vi "switch_load_1.vi"(0 "Node":string, 1 "event time":string="0.023560", 2 "Event type":string="BCG") -> (7 "Event switches":string caption="Result")   [LabVIEW 2019]
panel:
  in  "Evento?":bool
  # "CHAVEIA CARGAS DO SISTEMA"
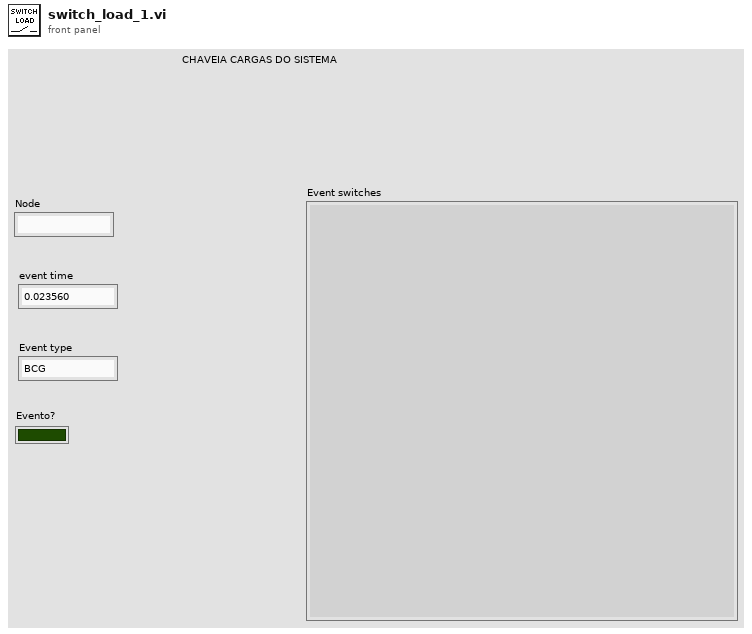
[diagram p1: front panel]
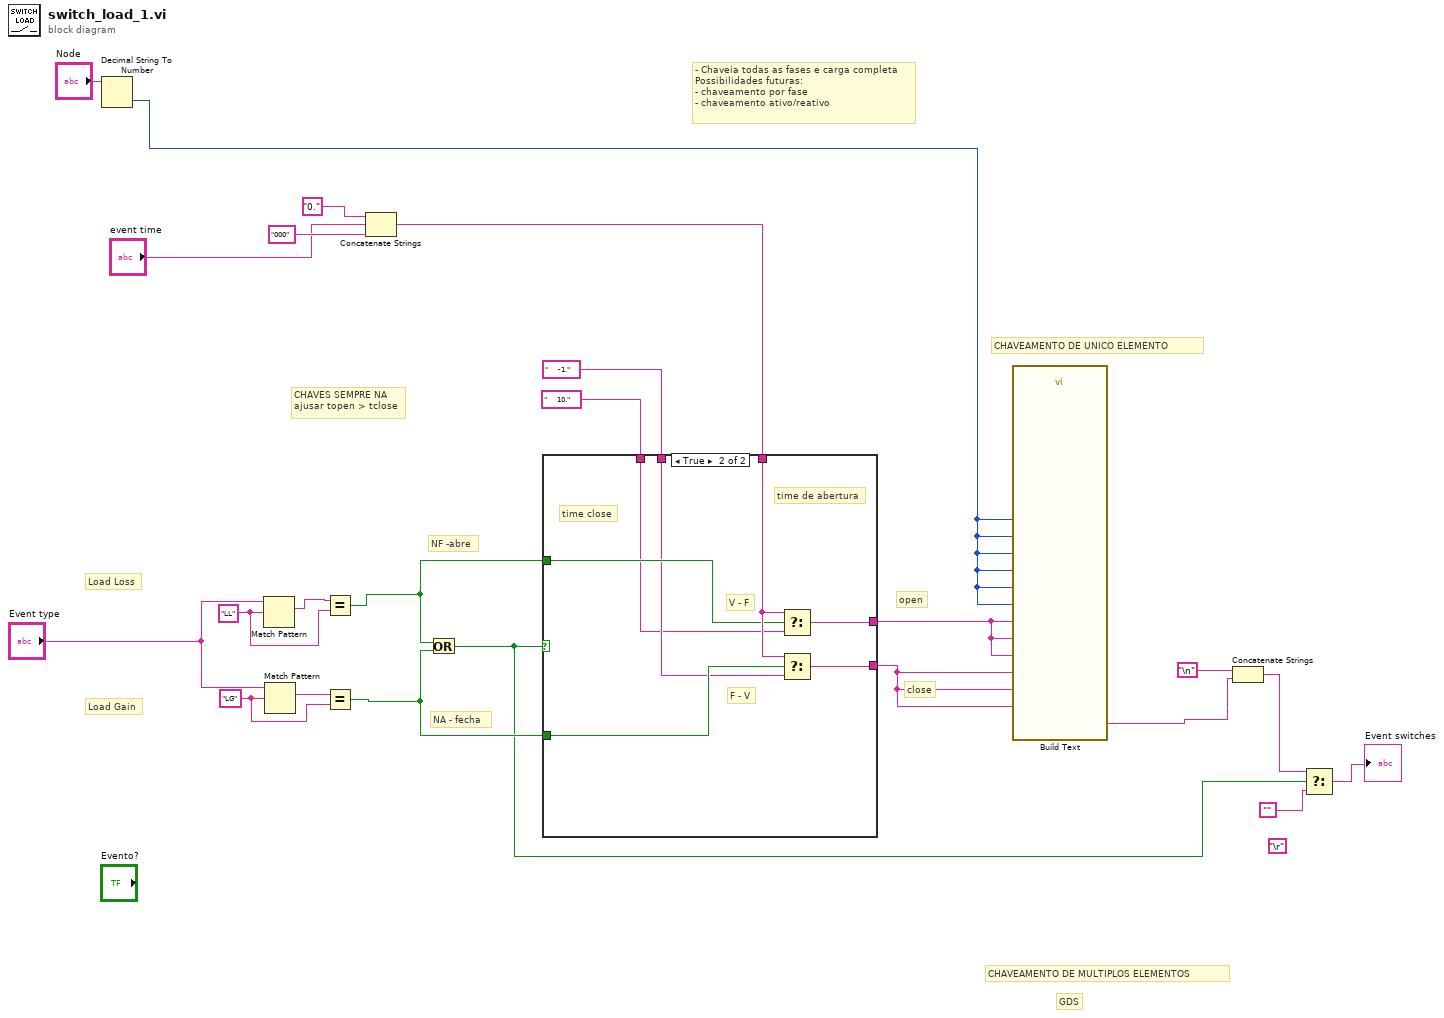
[diagram p0: block diagram]
diagram:
  (unwired) "\r"
  w18 = "LL" ("regular expression")
  w19 = "LG" ("regular expression")
  # "CHAVES SEMPRE NA\najusar topen > tclose"
  # "close"
  # "open"
  # "GDS"
  # "CHAVEAMENTO DE MULTIPLOS ELEMENTOS"
  # "CHAVEAMENTO DE UNICO ELEMENTO"
  # "NA - fecha"
  # "NF -abre"
  # "- Chaveia todas as fases e carga completa\nPossibilidades futuras:\n- chaveamento por fase\n- chaveamento ativo/reativo"
  # "Load Gain"
  # "Load Loss"
  n1 = Decimal String To Number(string="Node") -> (number=w11:i32)  [unwired: 2 in, 1 out]
  n2 = Match Pattern(string="Event type", regular expression=w18) -> (match substring=w17:string)  [unwired: 1 in, 3 out]
  n3 = Match Pattern(string="Event type", regular expression=w19) -> (match substring=w21:string)  [unwired: 1 in, 3 out]
  n4 = Equal?(x=w17, y=w18) -> (x = y?=w8:bool)
  n5 = Equal?(x=w21, y=w19) -> (x = y?=w7:bool)
  n6 = Concatenate Strings("0." ("string"), "event time", "000" ("string")) -> (w12:string)
  n7 = Or(x=w8, y=w7) -> (x .or. y?=w6:bool)
  n8 = case shown="True" w6 {
    tunnel: w12 -> [_ w32]
    tunnel: "     -1." -> [w25 w27]
    tunnel: "     10." -> [w24 w26]
    tunnel: [w25 w30] -> w9
    tunnel: [w24 w31] -> w10
    tunnel: w7 -> [_ w28]
    tunnel: w8 -> [_ w29]
    frame False {
    }
    frame True {
      # "F - V"
      # "V - F"
      # "time close"
      # "time de abertura"
      n9 = Select(t=w32, s=w29, f=w26) -> (s? t:f=w31:string)
      n10 = Select(t=w32, s=w28, f=w27) -> (s? t:f=w30:string)
    }
  }
  n11 = call "Build Text"("inA"=w11, "inA_2"=w11, "time_close_A"=w9, "time_open_A"=w10, "inB"=w11, "inB_2"=w11, "time_close_B"=w9, "time_open_B"=w10, "inC"=w11, "inC_2"=w11, "time_close_C"=w9, "time_open_C"=w10) -> ("Result"=w2:string)  [unwired: 14 in, 1 out]
  n12 = Concatenate Strings("\n", w2) -> (w1:string)
  n13 = Select(t=w1, s=w6, f="") -> (s? t:f=→"Event switches":string)
